vi "Send Current State Notification.vi"(8 "error in (no error)":errorcluster, 10 "State":refnum<class>, 11 "Context in":refnum<class "Context.lvclass">) -> (0 "error out":errorcluster, 3 "Context out":refnum<class "Context.lvclass">)   [LabVIEW 2024, in "Context.lvlib" / "Context.lvclass"]
uses:
  Context.lvclass
  Context.lvclass/Context.ctl
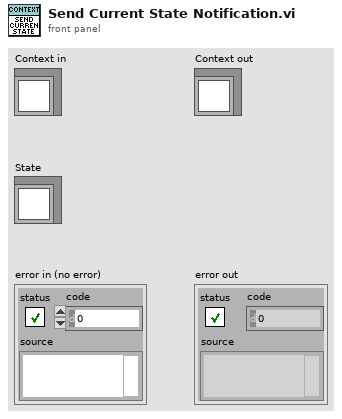
[diagram p1: front panel]
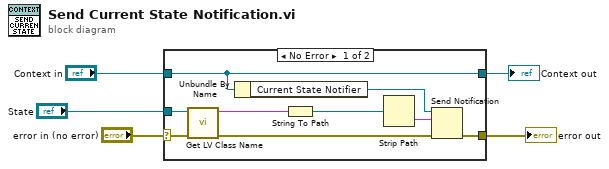
[diagram p0: block diagram]
diagram:
  n1 = case shown="No Error" "error in (no error)" {
    selector: "error in (no error)" -> [w11 w16]
    tunnel: [w9 w16] -> w4
    tunnel: [w14 w15] -> w2
    tunnel: "Context in" -> [w14 w15]
    tunnel: "State" -> [w12 _]
    frame No Error {
      n2 = call <vilib>:"Get LV Class Name.vi"("error in (no error)"=w11, "object"=w12) -> ("error out"=w10:errorcluster, "class name"=w8:string)  [unwired: 8 in]
      n3 = Unbundle By Name(w14) -> ("Current State Notifier"=w13:refnum<notifier>)
      n4 = String To Path(string=w8) -> (path=w7:path)
      n5 = Strip Path(path=w7) -> (name=w6:string)  [unwired: 1 out]
      n6 = Send Notification(notification=w6, notifier=w13, error in (no error)=w10) -> (error out=w9:errorcluster)  [unwired: 1 out]
    }
    frame Error {
    }
  }
  "error out" <- w4
  "Context out" <- w2
